vi "FTW-Probe-String.vi"(11 "Probe Value":string) -> (2 "Probe Value for Display":string, 3 "Breakpoint?":bool)   [LabVIEW 2015]
uses:
  src/regex/FTW-Regex-Execute.vi
  src/string/FTW-STR-ReplaceWhitespace.vi
  src/error/FTW-ERR-ThrowGenericError.vi
  src/error/FTW-ERR-Clear.vi
  src/regex/FTW-Regex-ReplaceAll.vi
  src/error/FTW-ERR-ThrowError.vi
  src/error/FTW-ERR-CallChain.vi
  src/error/FTW-ERR-NoErrorConstant.vi
  src/string/FTW-STR-Array-Delimit.vi
  src/regex/FTW-Regex-Construct.vi
  lib/FTW-KernelFilepath.vi
  src/regex/FTW-Regex-Destroy.vi
panel:
  in  "Pause on Regex Match?":bool
  in  "Regex to Match":string="(?six)"
  out "Regex Match":string
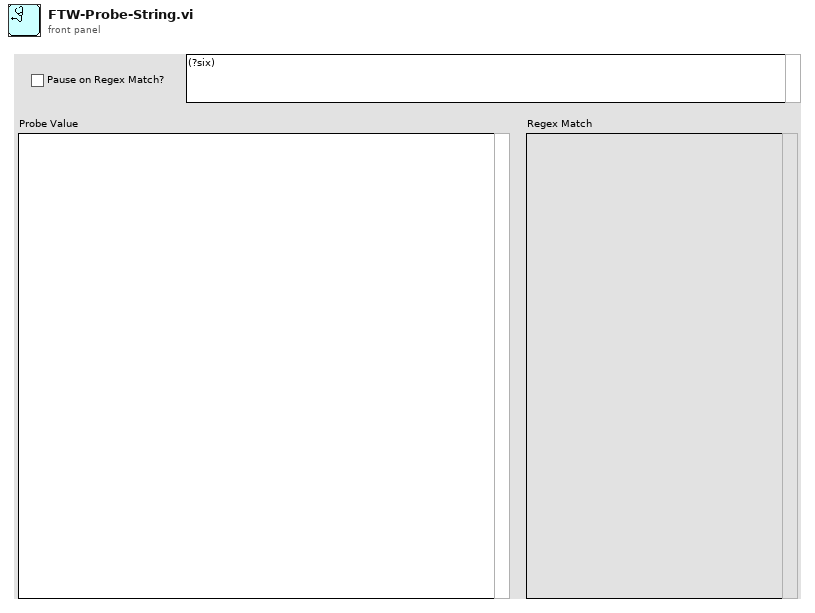
[diagram p1: front panel]
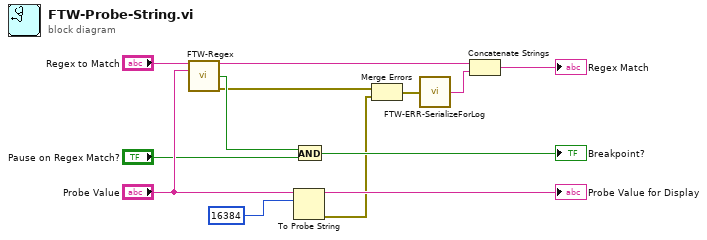
[diagram p0: block diagram]
diagram:
  n1 = call "FTW-Regex.vi"("Regular Expression"="Regex to Match", "Input String"="Probe Value") -> ("Match"=w6:string, "Match Found?"=w9:bool, "error out"=w3:errorcluster)  [unwired: 9 in, 2 out]
  n2 = To Probe String(6:u32 16384 ("maximum string length (1024)"), 7:"Probe Value") -> (0:w1:errorcluster, 3:→"Probe Value for Display":string)  [unwired: 1 in]
  n3 = And(x=w9, y="Pause on Regex Match?") -> (x .and. y?=→"Breakpoint?":bool)
  n4 = Merge Errors(w3, w1) -> (w2:errorcluster)
  n5 = call "FTW-ERR-SerializeForLog.vi"("error in"=w2) -> ("Serialized Error"=w5:string)
  n6 = Concatenate Strings(w6, w5) -> (→"Regex Match":string)
